vi "Read Table Headers.vi"(8 "error in":errorcluster, 11 "Table Ref in":refnum<vi>) -> (0 "error out":errorcluster, 1 "Column Headers":string[](array[string]), 2 "Interpret As Unicode (Columns)":bool, 3 "Table Ref out":refnum<vi>, 4 "Interpret As Unicode (Rows)":bool, 6 "Row Headers":string[](array[string]))   [LabVIEW 2020, in "G-Unicode.lvlib"]
uses:
  G-Unicode.lvlib
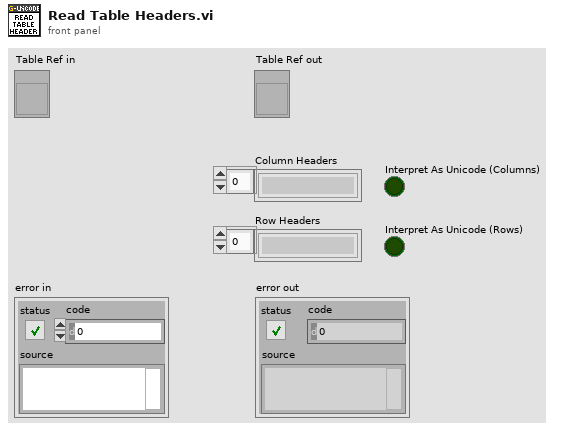
[diagram p1: front panel]
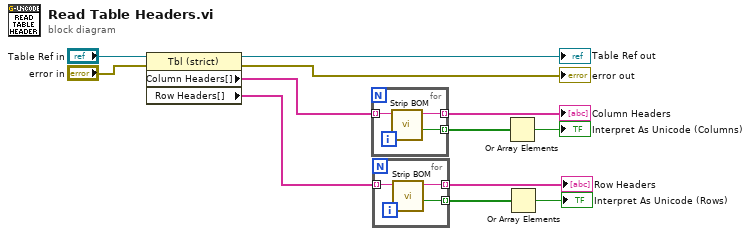
[diagram p0: block diagram]
diagram:
  n1 = property class="Tbl (strict)"(reference="Table Ref in", error in="error in") -> (reference out=→"Table Ref out":refnum<vi>, error out=→"error out":errorcluster, "Column Headers[]"=w7:string[], "Row Headers[]"=w5:string[])
  n2 = for {
    tunnel: w7 -> [w15] mode=indexing
    tunnel: [w14] -> w10 mode=indexing
    tunnel: [w13] -> w12 mode=indexing
    n3 = call "Strip BOM.vi"("String"=w15) -> ("BOM Found"=w13:bool, "String without BOM"=w14:string)  [unwired: 8 in, 1 out]
  }
  "Column Headers" <- w10
  n4 = for {
    tunnel: w5 -> [w18] mode=indexing
    tunnel: [w17] -> w3 mode=indexing
    tunnel: [w16] -> w6 mode=indexing
    n5 = call "Strip BOM.vi"("String"=w18) -> ("BOM Found"=w16:bool, "String without BOM"=w17:string)  [unwired: 8 in, 1 out]
  }
  "Row Headers" <- w3
  n6 = Or Array Elements(Boolean array=w12) -> (logical OR=→"Interpret As Unicode (Columns)":bool)
  n7 = Or Array Elements(Boolean array=w6) -> (logical OR=→"Interpret As Unicode (Rows)":bool)
